vi "VirtualDAQ_converter.vi"() -> ()   [LabVIEW 2019]
panel:
  in  "Base temperature":dbl(slide)=25.0 scale=0.0..100.0
  in  "Temperature spread":dbl(slide) scale=0.0..5.0
  in  "Ring":u16(ring) items=["Original Signal", "Convert to Voltage", "Convert to Temperature"]
  in  "Voltage":dbl(knob) scale=0.0..10.0
  out "Signal":dynamicdata(graph)
  in  "stop":bool
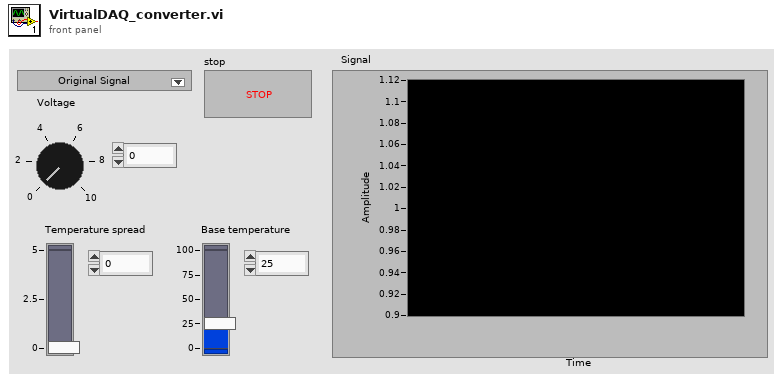
[diagram p1: front panel]
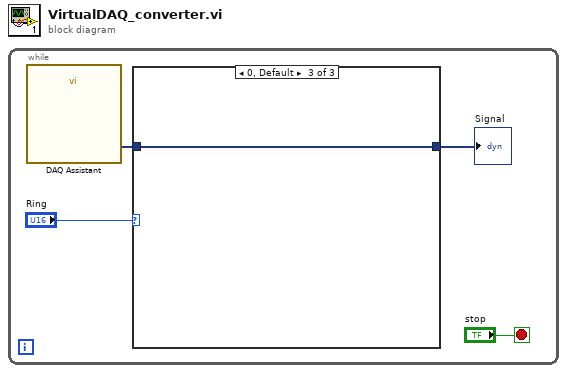
[diagram p0: block diagram]
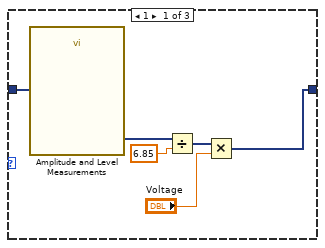
[diagram p2: hidden frame]
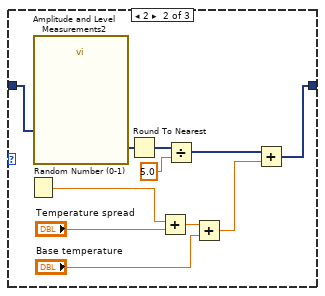
[diagram p3: hidden frame]
diagram:
  n1 = while {
    stop <- "stop" stop-if-true
    n2 = call "DAQ Assistant"() -> ("data"=w2:dynamicdata)  [unwired: 17 in, 2 out]
    n3 = case shown="0, Default" "Ring" {
      tunnel: w2 -> [w10 w20 w22]
      tunnel: [w7 w14 w22] -> w3
      frame 1 {
        n4 = call "Amplitude and Level Measurements"("Signals"=w10) -> ("RMS"=w6:dynamicdata)  [unwired: 13 in, 1 out]
        n5 = Divide(x=w6, y=6.85 ("x")) -> (x/y=w9:dynamicdata)
        n6 = Multiply(x=w9, y="Voltage") -> (x*y=w7:dynamicdata)
      }
      frame 2 {
        n7 = Random Number (0-1)() -> (number: 0 to 1=w16:dbl)
        n8 = call "Amplitude and Level Measurements2"("Signals"=w20) -> ("RMS"=w17:dynamicdata)  [unwired: 13 in, 1 out]
        n9 = Round To Nearest(number=w17) -> (nearest integer value=w19:dynamicdata)
        n10 = Add(x=w16, y="Temperature spread") -> (x+y=w13:dbl)
        n11 = Divide(x=w19, y=5.0) -> (x/y=w15:dynamicdata)
        n12 = Add(x=w13, y="Base temperature") -> (x+y=w11:dbl)
        n13 = Add(x=w15, y=w11) -> (x+y=w14:dynamicdata)
      }
      frame 0, Default {
      }
    }
    "Signal" <- w3
  }
